vi "open.vi"(0 "graph":cluster{"intrfrgrm":T1, "spectrum":T1}, 1 "virtualSource":bool, 2 "spectrIdx":u16, 3 "buffer size interferogram":i32, 4 "buffer size spectrum":i32=5000000 format="%^.0e", 5 "error in (no error)":errorcluster, 6 "plot zoom step factor":dbl=3.0 format="%.2f", 7 "peaks max nr (100)":u32=100, 8 "rel humidity (%)":dbl=50.0 format="%.2f", 9 "traces":T3={"nr interferogram (2)"=2, "nr spectrum (10)"=10}, 10 "spectrometer serial nr":string, 11 "FTSLV.dll folder":string, 12 "spectrometer model":string, 13 "OSA series":T2) -> (14 "duplicate reference":refnum<class "OSA.lvclass">, 19 "error out":errorcluster)   [LabVIEW 2010, in "OSA.lvclass"]
doc: "Lower level initialisation without readout of range/serial nr etc; might be useful when not having support vis located at default location."
uses:
  OSA.lvclass
  typeDef/OSA_series.ctl
  private/graph_intensity.ctl
  FTSLib.dll
  OSA20X_misc.lvlib
  _OSA200_class/OSA200.lvclass
  _OSA300_class/OSA300.lvclass
panel:
  in  "reference":refnum<class "OSA.lvclass">
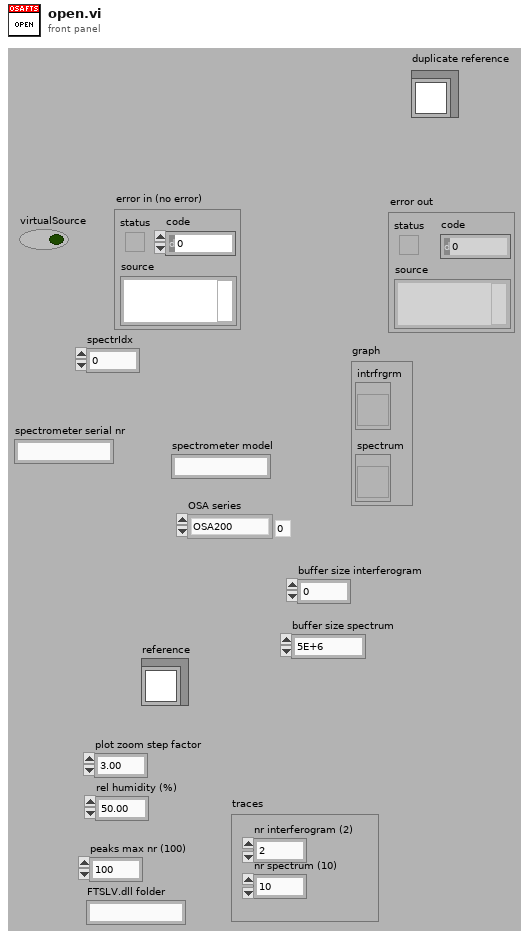
[diagram p1: front panel]
types:
  T1 = typedef "OSA.lvclass/graph_intensity.ctl" = refnum<vi>
  T2 = typedef "OSA.lvclass/OSA_series.ctl" = enum16{"OSA200", "OSA300", "UNKNOWN"}
  T3 = cluster{"nr interferogram (2)":i32, "nr spectrum (10)":i32}
  T4 = enum16{"get", "init", "set interferogram", "set spectrum", "cleanUp"}
  T5 = enum32{"invalid app kind", "Development System", "Run Time System", "Student Edition", "Embedded LabVIEW", "Evaluation", "Custom"}
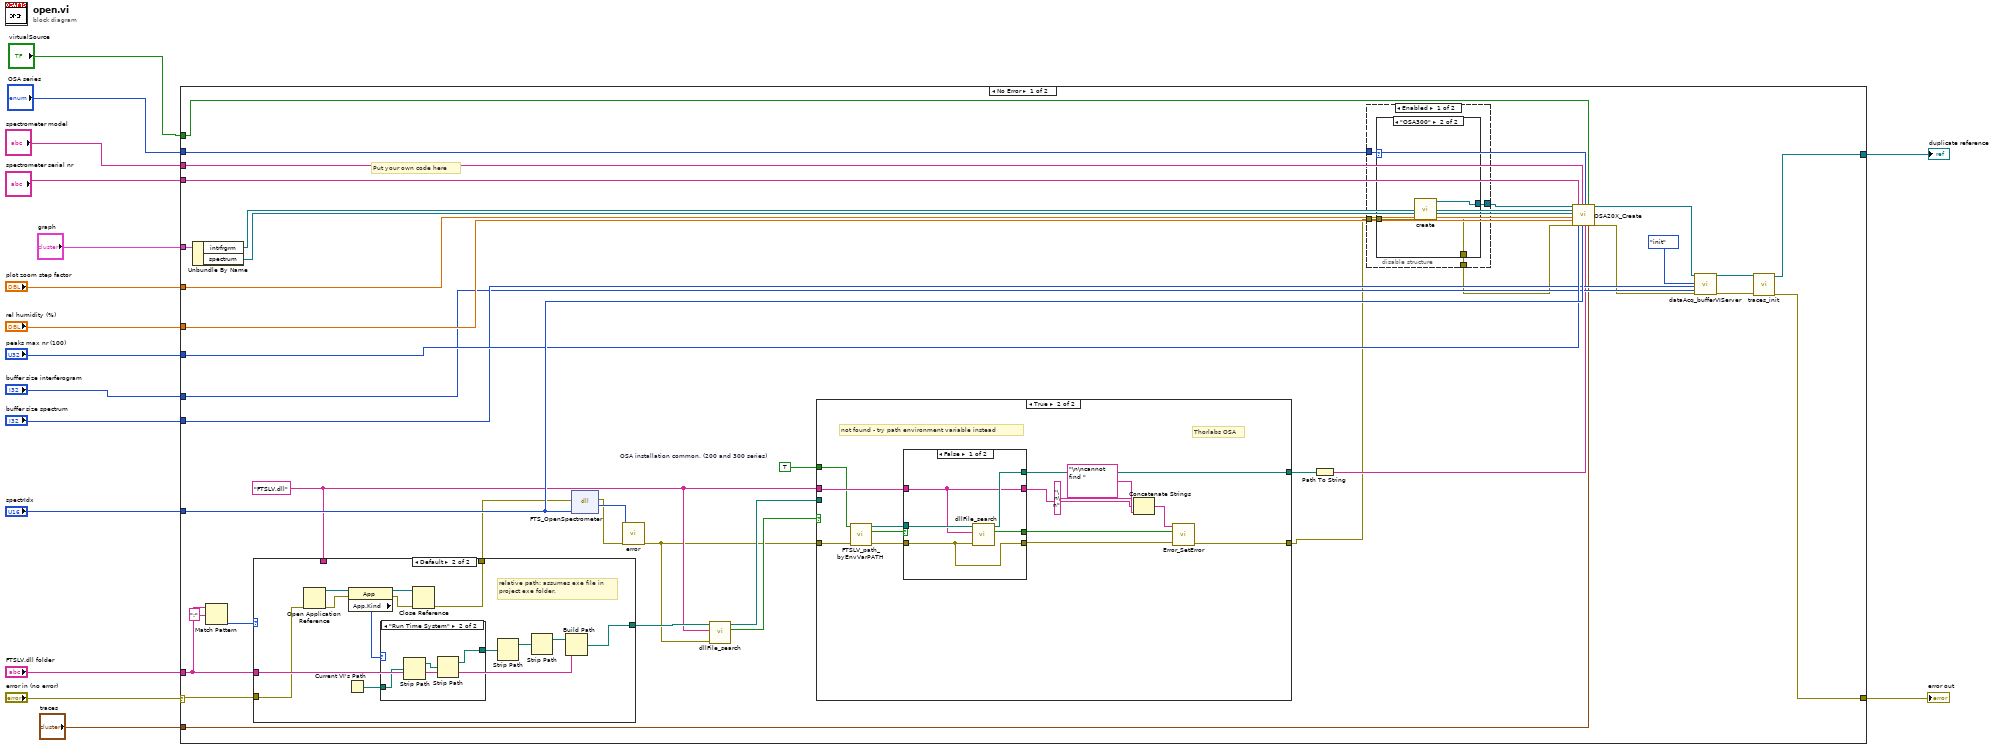
[diagram p0: block diagram]
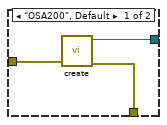
[diagram p2: hidden frame]
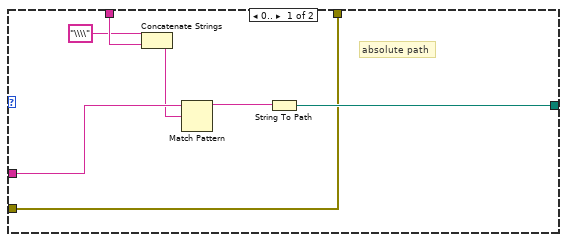
[diagram p4: hidden frame]
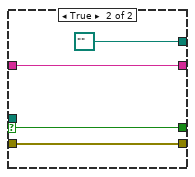
[diagram p7: hidden frame]
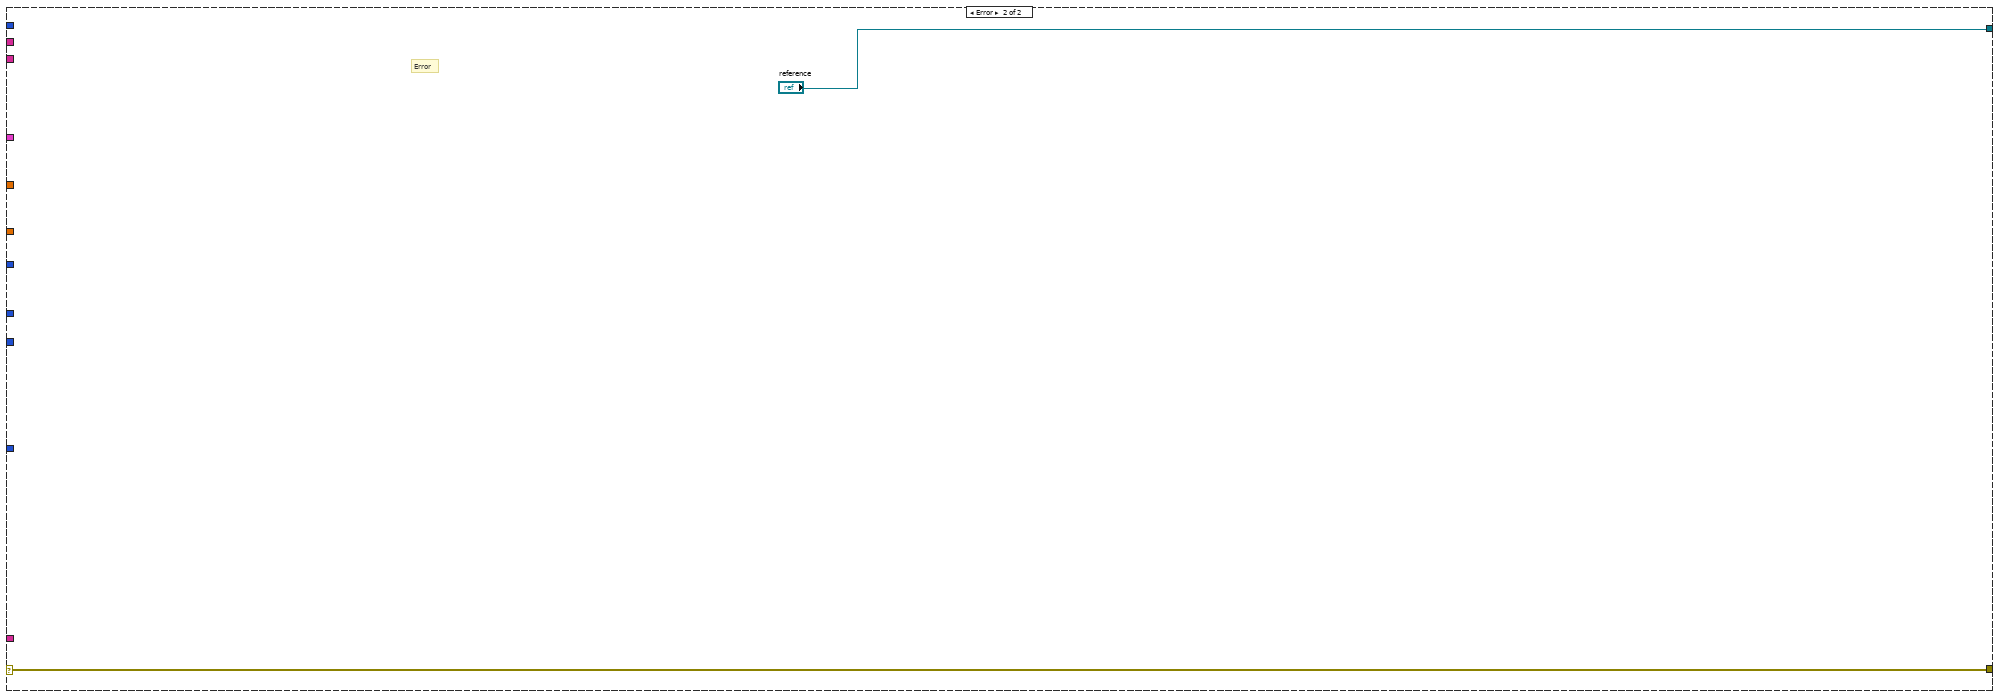
[diagram p8: hidden frame]
diagram:
  n1 = case shown="No Error" "error in (no error)" {
    selector: "error in (no error)" -> [w43 w116]
    tunnel: [w28 w116] -> w16
    tunnel: [w29 "reference"] -> w14
    tunnel: "spectrIdx" -> [w54 _]
    tunnel: "buffer size interferogram" -> [w47 _]
    tunnel: "plot zoom step factor" -> [w53 _]
    tunnel: "rel humidity (%)" -> [w52 _]
    tunnel: "peaks max nr (100)" -> [w51 _]
    tunnel: "FTSLV.dll folder" -> [w40 _]
    tunnel: "buffer size spectrum" -> [w48 _]
    tunnel: "spectrometer serial nr" -> [w46 _]
    tunnel: "spectrometer model" -> [w45 _]
    tunnel: "traces" -> [w32 _]
    tunnel: "OSA series" -> [w23 _]
    tunnel: "graph" -> [w27 _]
    tunnel: "virtualSource" -> [w17 _]
    frame No Error {
      w18 = TRUE  # OSA installation common, (200 and 300 series)
      w34 = "FTSLV.dll" ("element")
      # "Put your own code here"
      n2 = Unbundle By Name(w27) -> ("intrfrgrm"=w26:T1, "spectrum"=w25:T1)
      n3 = Match Pattern(string=w40, regular expression=":") -> (offset past match=w38:i32)  [unwired: 1 in, 3 out]
      n4 = case shown="Default" w38 {
        tunnel: w40 -> [w72 w85]
        tunnel: w43 -> [w69 w79]
        tunnel: [w69 w77] -> w42
        tunnel: [w70 w73] -> w37
        tunnel: w34 -> [w68 _]
        frame 0.. {
          # "absolute path"
          n5 = Concatenate Strings("\\\\" ("element"), w68) -> (w67:string)
          n6 = Match Pattern(string=w72, regular expression=w67) -> (before substring=w71:string)  [unwired: 1 in, 3 out]
          n7 = String To Path(string=w71) -> (path=w70:path)
        }
        frame Default {
          # "relative path: assumes exe file in\nproject exe folder."
          n8 = Open Application Reference(8:w79) -> (0:w83:errorcluster, 3:w82:refnum<vi>)  [unwired: 3 in]
          n9 = Current VI's Path() -> (path=w76:path)
          n10 = property class="App"(reference=w82, error in=w83) -> (reference out=w84:refnum<vi>, error out=w80:errorcluster, "App.Kind"=w74:T5)
          n11 = case shown="\"Run Time System\"" w74 {
            tunnel: w76 -> [w86 w88]
            tunnel: [w86 w89] -> w75
            frame "invalid app kind", Default {
            }
            frame "Run Time System" {
              n12 = Strip Path(path=w88) -> (stripped path=w87:path)  [unwired: 1 out]
              n13 = Strip Path(path=w87) -> (stripped path=w89:path)  [unwired: 1 out]
            }
          }
          n14 = Close Reference(reference=w84, error in (no error)=w80) -> (error out=w77:errorcluster)
          n15 = Strip Path(path=w75) -> (stripped path=w78:path)  [unwired: 1 out]
          n16 = Strip Path(path=w78) -> (stripped path=w81:path)  [unwired: 1 out]
          n17 = Build Path(base path=w81, name or relative path=w85) -> (appended path=w73:path)
        }
      }
      n18 = dll-call lib="FTSLib.dll" fn="FTS_OpenSpectrometer"(error in=w42, "spectrIdx"=w54) -> (error out=w44:errorcluster, "return type"=w55:i32)  [unwired: 3 in, 1 out]
      n19 = call "error.vi"("result code"=w55, "error in (no error)"=w44) -> ("error out"=w33:errorcluster)  [unwired: 15 in, 2 out]
      n20 = call "dllFile_search.vi"("error in (no error)"=w33, "file search"=w34, "search root"=w37) -> ("notFound"=w36:bool, "Path"=w35:path)  [unwired: 6 in, 1 out]
      n21 = case shown="True" w36 {
        tunnel: w35 -> [w91 _]
        tunnel: [w91 w102] -> w50
        tunnel: w34 -> [_ w101]
        tunnel: w33 -> [w90 w105]
        tunnel: [w90 w95] -> w24
        tunnel: w18 -> [_ w92]
        frame False {
          # "File found by parameter input"
        }
        frame True {
          # "Thorlabs OSA"
          # "not found - try path environment variable instead"
          n22 = call "FTSLV_path_byEnvVarPATH.vi"("error in (no error)"=w105, "OSA installation common, (200 and 300 series)"=w92) -> ("error out"=w103:errorcluster, "not found"=w94:bool, "Thorlabs OSA path"=w104:path)  [unwired: 7 in]
          n23 = case shown="False" w94 {
            selector: w94 -> [_ w111]
            tunnel: w104 -> [w110 _]
            tunnel: w103 -> [w106 w113]
            tunnel: [w109 path ""] -> w102
            tunnel: [w106 w113] -> w96
            tunnel: w101 -> [w108 w112]
            tunnel: [w108 w112] -> w97
            tunnel: [w107 w111] -> w93
            frame False {
              n24 = call "dllFile_search.vi"("error in (no error)"=w106, "file search"=w108, "search root"=w110) -> ("notFound"=w107:bool, "Path"=w109:path)  [unwired: 6 in, 1 out]
            }
            frame True {
            }
          }
          n25 = Concatenate Strings("\n\ncannot find " ("string"), w97, "\n\n" ("string")) -> (w100:string)
          n26 = call "Error_SetError.vi"("error in"=w96, "status (true)"=w93, "source(\"\")"=w100) -> ("error out"=w95:errorcluster)  [unwired: 4 in]
        }
      }
      n27 = Path To String(path=w50) -> (string=w41:string)
      n28 = disable-structure shown="Enabled" {
        disable-tunnel: [w59 _] -> w22
        disable-tunnel: w24 -> [w58 _]
        disable-tunnel: [w57 _] -> w20
        disable-tunnel: w23 -> [w56 _]
        frame Enabled {
          n29 = case shown="\"OSA300\"" w56 {
            tunnel: [w60 w63] -> w59
            tunnel: w58 -> [w62 w65]
            tunnel: [w61 w64] -> w57
            frame "OSA200", Default {
              n30 = call "create.vi"("error in (no error)"=w62) -> ("error out"=w61:errorcluster, "OSA200.lvclass"=w60:refnum<class "OSA200.lvclass">)  [unwired: 9 in]
            }
            frame "OSA300" {
              n31 = call "create.vi"("error in (no error)"=w65) -> ("error out"=w64:errorcluster, "OSA300 out"=w63:refnum<class "OSA300.lvclass">)  [unwired: 9 in]
            }
          }
        }
        frame Disabled {
        }
      }
      n32 = call "OSA20X_Create.vi"("reference in"=w22, "Graph Intrfrgrm"=w26, "Graph Spectrum"=w25, "plot zoom step factor"=w53, "rel humidity (50%)"=w52, "error in (no error)"=w20, "spectrometer serial nr"=w46, "peaks max nr (100)"=w51, "spectrometer model"=w45, "spectrometerIdx"=w54, "OSA series"=w23, "path FTSLV.dll"=w41, "virtualSource"=w17, "traces"=w32) -> ("reference"=w21:refnum<class "OSA.lvclass">, "error out"=w19:errorcluster)  [unwired: 4 in]
      n33 = call "dataAcq_bufferVIServer.vi"("reference"=w21, "action"=T4."init", "bufferSize spectrum"=w48, "bufferSize interferogram"=w47, "error in (no error)"=w19) -> ("duplicate reference"=w30:refnum<class "OSA.lvclass">, "error out"=w31:errorcluster)  [unwired: 7 in, 6 out]
      n34 = call "traces_init.vi"("reference"=w30, "error in (no error)"=w31) -> ("duplicate reference"=w29:refnum<class "OSA.lvclass">, "error out"=w28:errorcluster)  [unwired: 16 in]
    }
    frame Error {
      # "Error"
    }
  }
  "error out" <- w16
  "duplicate reference" <- w14
